vi "range.vi"(0 "size":i32, 5 "index":i32) -> (4 "lower limit":i32)   [LabVIEW 2019]
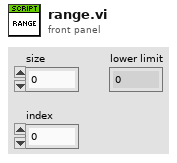
[diagram p1: front panel]
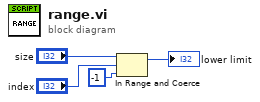
[diagram p0: block diagram]
diagram:
  n1 = In Range and Coerce(upper limit="size", x="index", lower limit=-1) -> (coerced(x)=→"lower limit":i32)  [unwired: 1 out]
